vi "swerve_periodic_trajlib.vi"(11 "in ModuleStates":T1[](array[typedef]) {"Angle"."SIN" format="%13.4f"; "Angle"."COS" format="%13.4f"; "Angle"."VALUE" format="%13.4f"}) -> ()   [LabVIEW 2020]
uses:
  <vilib>/Rock Robotics/WPI/ThirdParty/JAS_Junk/TrajLib/SWERVE_DRIVE_MODULE_STATE.ctl
  <vilib>/Rock Robotics/WPI/ThirdParty/JAS_Junk/TrajLib/ROTATION2D.ctl
  <vilib>/Rock Robotics/WPI/ThirdParty/Phoenix-LabVIEW/Motor Controller/Controls/CTRE_Phoenix_MotorControl_ControlMode.ctl
  <vilib>/Rock Robotics/WPI/ThirdParty/JAS_Junk/TrajLib/Conv_Radians_Deg.vi
  swerve_globals.vi
  <vilib>/Rock Robotics/WPI/ThirdParty/Phoenix-LabVIEW/Motor Controller/Get/CTRE_Phoenix_MotorController_GetSelectedSensorData.vi
  TitanLib/Lib/TitanLib.lvlib
  <vilib>/Rock Robotics/WPI/ThirdParty/JAS_Junk/TrajLib/Trajectory_Library.lvlib
panel:
  in  "Drive Motor Constants":T3
  in  "Set Drive Constants":bool
  in  "Set Azimuth Constants":bool
  in  "Azimuth Constants":T3
  out "Pose Estimation (in)":cluster{"Pose[0]":dbl, "Pose[1]":dbl}[](graph)
  in  "wheel offset (in)":dbl format="%_6g"
  in  "Reset Odometry?":bool
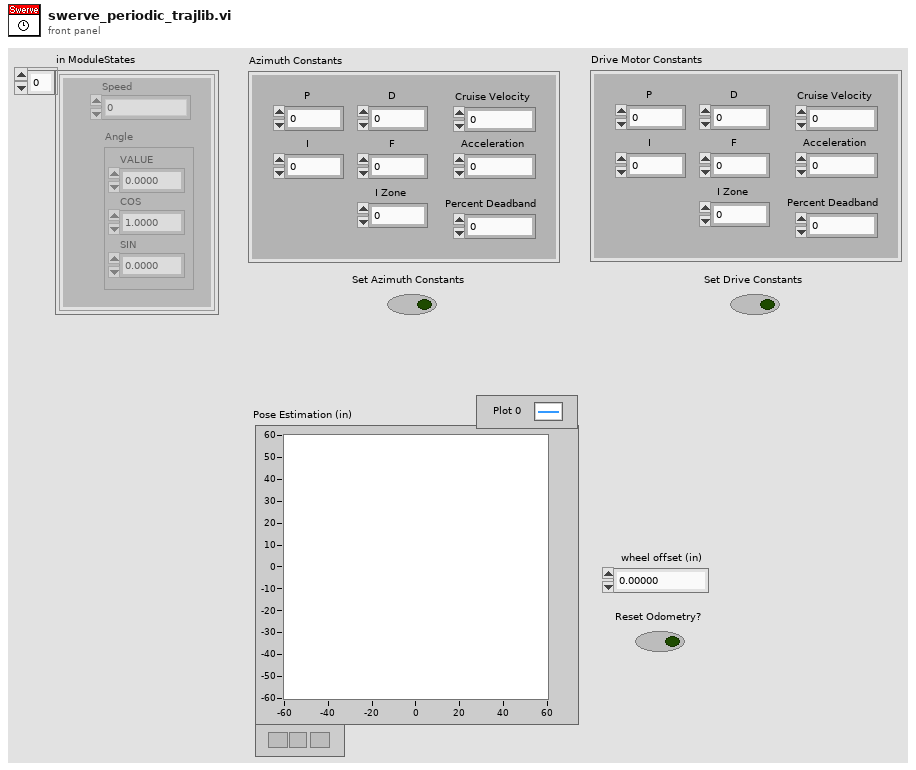
[diagram p1: front panel]
types:
  T1 = typedef "Trajectory_Library.lvlib/SWERVE_DRIVE_MODULE_STATE.ctl" = cluster{"Speed":dbl, "Angle":T2}
  T2 = typedef "Trajectory_Library.lvlib/ROTATION2D.ctl" = cluster{"VALUE":dbl, "COS":dbl, "SIN":dbl}
  T3 = cluster{"P":dbl, "I":dbl, "D":dbl, "F":dbl, "I Zone":dbl, "Cruise Velocity":i32, "Acceleration":i32, "Percent Deadband":dbl}
  T4 = typedef "CTRE_Phoenix_MotorControl_ControlMode.ctl" = u16
  T5 = typedef "WPI_MotorControlDeviceRef.ctl" = cluster{"DeviceStatus":errorcluster, "Type":T6, "PWM":cluster{"PWM Channel":T7, "DeadBand":T8}, "CAN":cluster{"Device Number":u8, "SetOutput VI Ref":variant, "GetOutput VI Ref":variant, "Enable VI Ref":variant, "Disable VI Ref":variant, "Data":variant}, "Invert":bool, "DIO PWM":cluster{"PWM \"Enable\" Channel":T7, "DIOChannel":T9, "PWM Rate":dbl}}
  T6 = typedef "WPI_MotorControlType.ctl" = enum16{"PWM", "CAN", "DIO PWM"}
  T7 = typedef "FPGA_DIOPWMChannel.ctl" = enum8{"PWM 0", "PWM 1", "PWM 2", "PWM 3", "PWM 4", "PWM 5", "PWM 6", "PWM 7", "PWM 8", "PWM 9", "PWM MXP 0", "PWM MXP 1", "PWM MXP 2", "PWM MXP 3", "PWM MXP 4", "PWM MXP 5", "PWM MXP 6", "PWM MXP 7", "PWM MXP 8", "PWM MXP 9", "Invalid"}
  T8 = typedef "WPI_PWMDeadband.ctl" = cluster{"Name":string, "maxPositivePwm":i32, "minPositivePwm":i32, "centerPwm":i32, "maxNegativePwm":i32, "minNegativePwm":i32, "angularRange":u16}
  T9 = typedef "FPGA_DIOChannel.ctl" = enum8{"DIO 0", "DIO 1", "DIO 2", "DIO 3", "DIO 4", "DIO 5", "DIO 6", "DIO 7", "DIO 8", "DIO 9", "DIO MXP 0", "DIO MXP 1", "DIO MXP 2", "DIO MXP 3", "DIO MXP 4", "DIO MXP 5", "DIO MXP 6", "DIO MXP 7", "DIO MXP 8", "DIO MXP 9", "DIO MXP 10", "DIO MXP 11", "DIO MXP 12", "DIO MXP 13", "DIO MXP 14", "DIO MXP 15", "SPI Port CS1", "SPI Port CS2", "SPI Port CS3", "SPI Port MISO", "SPI Port MOSI", "Invalid"}
  T10 = typedef "NI_Matrix.lvlib/RealMatrix.ctl" = dbl[][]
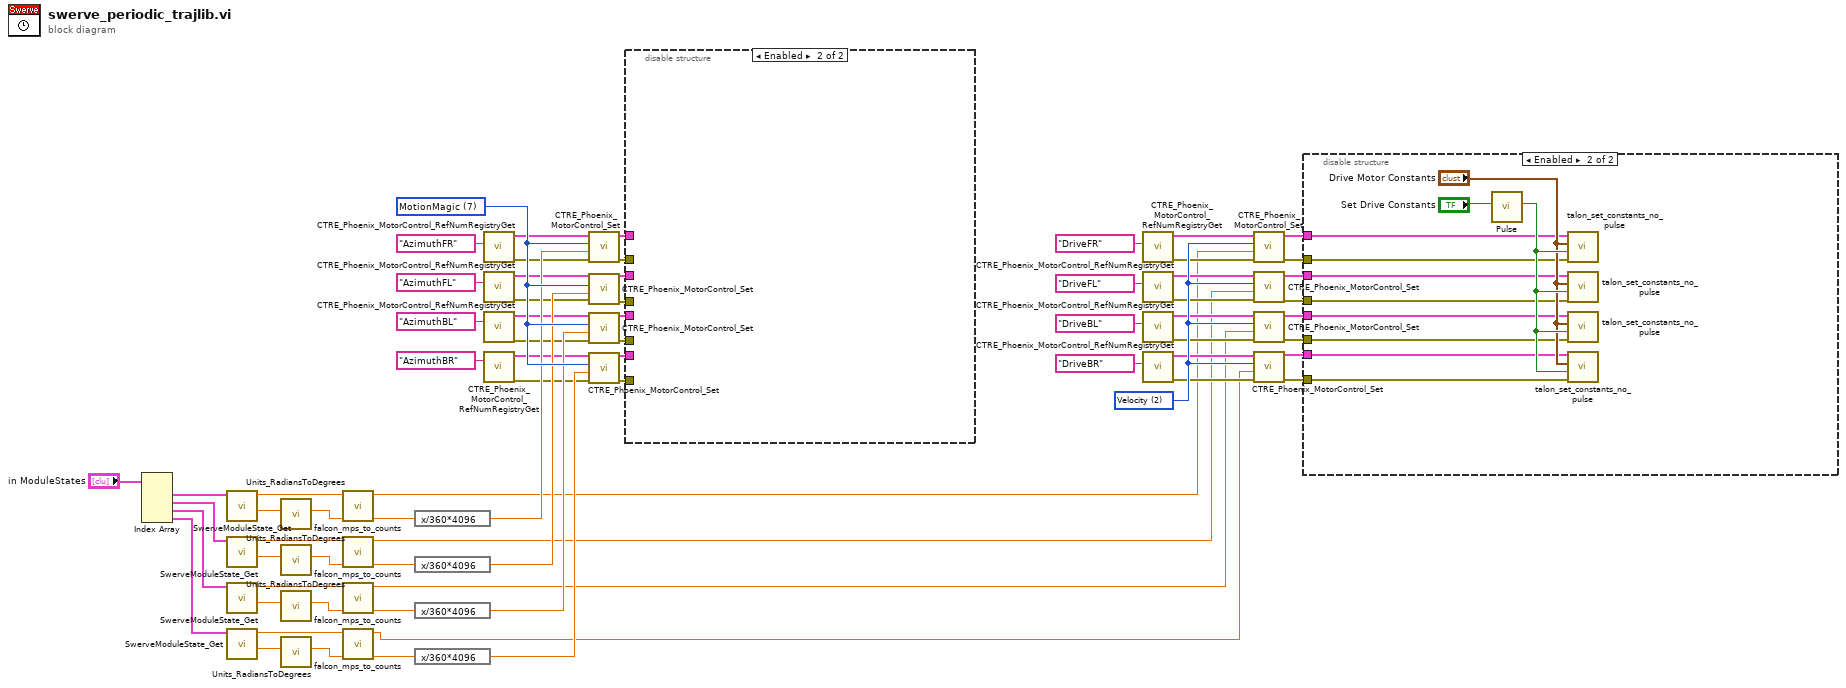
[diagram p0: block diagram]
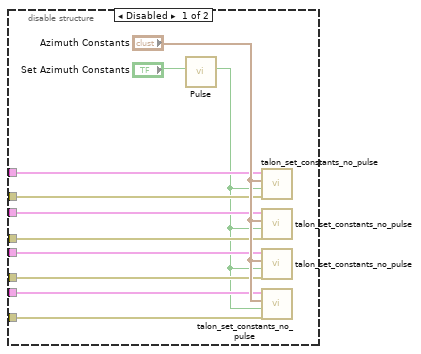
[diagram p2: hidden frame]
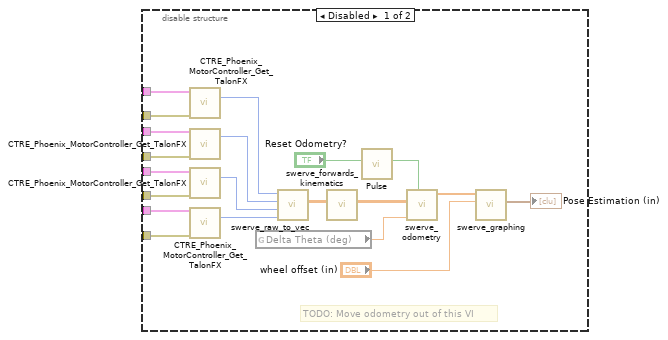
[diagram p3: hidden frame]
diagram:
  w62 = T4 2 items=["PercentOutput"=0, "Position"=1, "Velocity"=2, "Current"=3, "Follower"=5, "MotionProfile"=6, "MotionMagic"=7, "MotionProfileArc"=10, "Disabled"=15] ("Control Mode")
  w67 = T4 7 items=["PercentOutput"=0, "Position"=1, "Velocity"=2, "Current"=3, "Follower"=5, "MotionProfile"=6, "MotionMagic"=7, "MotionProfileArc"=10, "Disabled"=15] ("Control Mode")
  n1 = Index Array(array="in ModuleStates") -> (element #1=w5:T1, element #2=w3:T1, element #3=w2:T1, element #4=w1:T1)  [unwired: 4 in]
  n2 = call <vilib>:"SwerveModuleState_Get.vi"("Desired State"=w5) -> ("Angle RADIANS"=w21:dbl, "Speed M/S"=w14:dbl)  [unwired: 9 in]
  n3 = call <vilib>:"SwerveModuleState_Get.vi"("Desired State"=w3) -> ("Angle RADIANS"=w18:dbl, "Speed M/S"=w15:dbl)  [unwired: 9 in]
  n4 = call <vilib>:"SwerveModuleState_Get.vi"("Desired State"=w2) -> ("Angle RADIANS"=w19:dbl, "Speed M/S"=w16:dbl)  [unwired: 9 in]
  n5 = call <vilib>:"SwerveModuleState_Get.vi"("Desired State"=w1) -> ("Angle RADIANS"=w20:dbl, "Speed M/S"=w17:dbl)  [unwired: 9 in]
  n6 = call <vilib>:"Units_RadiansToDegrees.vi"("Radians"=w21) -> ("Degrees"=w13:dbl)  [unwired: 10 in]
  n7 = call <vilib>:"Units_RadiansToDegrees.vi"("Radians"=w18) -> ("Degrees"=w12:dbl)  [unwired: 10 in]
  n8 = call <vilib>:"Units_RadiansToDegrees.vi"("Radians"=w19) -> ("Degrees"=w11:dbl)  [unwired: 10 in]
  n9 = call <vilib>:"Units_RadiansToDegrees.vi"("Radians"=w20) -> ("Degrees"=w10:dbl)  [unwired: 10 in]
  n10 = call "falcon_mps_to_counts.vi"("Velocity (m/s)"=w14) -> ("Velocity (Counts/100ms)"=w9:dbl)  [unwired: 10 in]
  n11 = call "falcon_mps_to_counts.vi"("Velocity (m/s)"=w15) -> ("Velocity (Counts/100ms)"=w8:dbl)  [unwired: 10 in]
  n12 = call "falcon_mps_to_counts.vi"("Velocity (m/s)"=w16) -> ("Velocity (Counts/100ms)"=w7:dbl)  [unwired: 10 in]
  n13 = call "falcon_mps_to_counts.vi"("Velocity (m/s)"=w17) -> ("Velocity (Counts/100ms)"=w6:dbl)  [unwired: 10 in]
  n14 = expression code="x/360*4096"(w13) -> (w66:dbl)
  n15 = expression code="x/360*4096"(w12) -> (w65:dbl)
  n16 = expression code="x/360*4096"(w11) -> (w64:dbl)
  n17 = expression code="x/360*4096"(w10) -> (w63:dbl)
  n18 = call <vilib>:"CTRE_Phoenix_MotorControl_RefNumRegistryGet.vi"("refnum name"="AzimuthFR") -> ("error out"=w48:errorcluster, "PhoenixMotorControlDevRef"=w49:T5)  [unwired: 9 in]
  n19 = call <vilib>:"CTRE_Phoenix_MotorControl_RefNumRegistryGet.vi"("refnum name"="AzimuthFL") -> ("error out"=w46:errorcluster, "PhoenixMotorControlDevRef"=w47:T5)  [unwired: 9 in]
  n20 = call <vilib>:"CTRE_Phoenix_MotorControl_RefNumRegistryGet.vi"("refnum name"="AzimuthBL") -> ("error out"=w44:errorcluster, "PhoenixMotorControlDevRef"=w45:T5)  [unwired: 9 in]
  n21 = call <vilib>:"CTRE_Phoenix_MotorControl_RefNumRegistryGet.vi"("refnum name"="AzimuthBR") -> ("error out"=w42:errorcluster, "PhoenixMotorControlDevRef"=w43:T5)  [unwired: 9 in]
  n22 = call <vilib>:"CTRE_Phoenix_MotorControl_Set.vi"("error in (no error)"=w48, "Output"=w66, "Control Mode"=w67, "PhoenixMotorControlDevRef"=w49) -> ("error out"=w28:errorcluster, "PhoenixMotorControlDevRef"=w29:T5)  [unwired: 6 in]
  n23 = call <vilib>:"CTRE_Phoenix_MotorControl_Set.vi"("error in (no error)"=w46, "Output"=w65, "Control Mode"=w67, "PhoenixMotorControlDevRef"=w47) -> ("error out"=w26:errorcluster, "PhoenixMotorControlDevRef"=w27:T5)  [unwired: 6 in]
  n24 = call <vilib>:"CTRE_Phoenix_MotorControl_Set.vi"("error in (no error)"=w44, "Output"=w64, "Control Mode"=w67, "PhoenixMotorControlDevRef"=w45) -> ("error out"=w24:errorcluster, "PhoenixMotorControlDevRef"=w25:T5)  [unwired: 6 in]
  n25 = call <vilib>:"CTRE_Phoenix_MotorControl_Set.vi"("error in (no error)"=w42, "Output"=w63, "Control Mode"=w67, "PhoenixMotorControlDevRef"=w43) -> ("error out"=w22:errorcluster, "PhoenixMotorControlDevRef"=w23:T5)  [unwired: 6 in]
  n26 = disable-structure shown="Enabled" {
    disable-tunnel: w29 -> [w77 _]
    disable-tunnel: w28 -> [w76 _]
    disable-tunnel: w27 -> [w75 _]
    disable-tunnel: w26 -> [w74 _]
    disable-tunnel: w25 -> [w73 _]
    disable-tunnel: w24 -> [w72 _]
    disable-tunnel: w23 -> [w71 _]
    disable-tunnel: w22 -> [w70 _]
    frame Disabled {
      n27 = call "Pulse.vi"("Input"="Set Azimuth Constants") -> ("Output"=w68:bool)  [unwired: 10 in]
      n28 = call "talon_set_constants_no_pulse.vi"("error in"=w76, "Set Constants"=w68, "Constants"="Azimuth Constants", "PhoenixMotorControlDevRef"=w77) -> ()  [unwired: 6 in, 2 out]
      n29 = call "talon_set_constants_no_pulse.vi"("error in"=w74, "Set Constants"=w68, "Constants"="Azimuth Constants", "PhoenixMotorControlDevRef"=w75) -> ()  [unwired: 6 in, 2 out]
      n30 = call "talon_set_constants_no_pulse.vi"("error in"=w72, "Set Constants"=w68, "Constants"="Azimuth Constants", "PhoenixMotorControlDevRef"=w73) -> ()  [unwired: 6 in, 2 out]
      n31 = call "talon_set_constants_no_pulse.vi"("error in"=w70, "Set Constants"=w68, "Constants"="Azimuth Constants", "PhoenixMotorControlDevRef"=w71) -> ()  [unwired: 6 in, 2 out]
    }
    frame Enabled {
    }
  }
  n32 = call <vilib>:"CTRE_Phoenix_MotorControl_RefNumRegistryGet.vi"("refnum name"="DriveFR") -> ("error out"=w30:errorcluster, "PhoenixMotorControlDevRef"=w31:T5)  [unwired: 9 in]
  n33 = call <vilib>:"CTRE_Phoenix_MotorControl_RefNumRegistryGet.vi"("refnum name"="DriveFL") -> ("error out"=w32:errorcluster, "PhoenixMotorControlDevRef"=w33:T5)  [unwired: 9 in]
  n34 = call <vilib>:"CTRE_Phoenix_MotorControl_RefNumRegistryGet.vi"("refnum name"="DriveBL") -> ("error out"=w34:errorcluster, "PhoenixMotorControlDevRef"=w35:T5)  [unwired: 9 in]
  n35 = call <vilib>:"CTRE_Phoenix_MotorControl_RefNumRegistryGet.vi"("refnum name"="DriveBR") -> ("error out"=w36:errorcluster, "PhoenixMotorControlDevRef"=w37:T5)  [unwired: 9 in]
  n36 = call <vilib>:"CTRE_Phoenix_MotorControl_Set.vi"("error in (no error)"=w30, "Output"=w9, "Control Mode"=w62, "PhoenixMotorControlDevRef"=w31) -> ("error out"=w60:errorcluster, "PhoenixMotorControlDevRef"=w61:T5)  [unwired: 6 in]
  n37 = call <vilib>:"CTRE_Phoenix_MotorControl_Set.vi"("error in (no error)"=w32, "Output"=w8, "Control Mode"=w62, "PhoenixMotorControlDevRef"=w33) -> ("error out"=w58:errorcluster, "PhoenixMotorControlDevRef"=w59:T5)  [unwired: 6 in]
  n38 = call <vilib>:"CTRE_Phoenix_MotorControl_Set.vi"("error in (no error)"=w34, "Output"=w7, "Control Mode"=w62, "PhoenixMotorControlDevRef"=w35) -> ("error out"=w56:errorcluster, "PhoenixMotorControlDevRef"=w57:T5)  [unwired: 6 in]
  n39 = call <vilib>:"CTRE_Phoenix_MotorControl_Set.vi"("error in (no error)"=w36, "Output"=w6, "Control Mode"=w62, "PhoenixMotorControlDevRef"=w37) -> ("error out"=w54:errorcluster, "PhoenixMotorControlDevRef"=w55:T5)  [unwired: 6 in]
  n40 = disable-structure shown="Enabled" {
    disable-tunnel: w61 -> [w98 w106]
    disable-tunnel: w60 -> [w97 w105]
    disable-tunnel: w59 -> [w96 w104]
    disable-tunnel: w58 -> [w95 w103]
    disable-tunnel: w57 -> [w94 w99]
    disable-tunnel: w56 -> [w93 w102]
    disable-tunnel: w55 -> [w92 w101]
    disable-tunnel: w54 -> [w91 w100]
    frame Disabled {
      # "TODO: Move odometry out of this VI"
      n41 = call-poly <vilib>:"CTRE_Phoenix_MotorController_Get_TalonFX.vi"("PhoenixMotorControlDevRef"=w98, "error in"=w97) -> ("Position (Raw Sensor Units)"=w89:i32)  [unwired: 10 in, 3 out]
      n42 = call-poly <vilib>:"CTRE_Phoenix_MotorController_Get_TalonFX.vi"("PhoenixMotorControlDevRef"=w96, "error in"=w95) -> ("Position (Raw Sensor Units)"=w88:i32)  [unwired: 10 in, 3 out]
      n43 = call-poly <vilib>:"CTRE_Phoenix_MotorController_Get_TalonFX.vi"("PhoenixMotorControlDevRef"=w94, "error in"=w93) -> ("Position (Raw Sensor Units)"=w87:i32)  [unwired: 10 in, 3 out]
      n44 = call-poly <vilib>:"CTRE_Phoenix_MotorController_Get_TalonFX.vi"("PhoenixMotorControlDevRef"=w92, "error in"=w91) -> ("Position (Raw Sensor Units)"=w82:i32)  [unwired: 10 in, 3 out]
      n45 = global read "swerve_globals.vi" "Delta Theta (deg)"() -> (w83:dbl)
      n46 = call "swerve_raw_to_vec.vi"("Raw Position BR"=w82, "Raw Position BL"=w87, "Raw Position FL"=w88, "Raw Position FR"=w89) -> ("Output Vector"=w81:T10)  [unwired: 7 in]
      n47 = call "swerve_forwards_kinematics.vi"("Input Vector"=w81) -> ("Output Vector"=w86:T10)  [unwired: 10 in]
      n48 = call "Pulse.vi"("Input"="Reset Odometry?") -> ("Output"=w79:bool)  [unwired: 10 in]
      n49 = call "swerve_odometry.vi"("Reset?"=w79, "Delta Theta (deg)"=w83, "input vector"=w86) -> ("Pose"=w85:dbl[])  [unwired: 8 in]
      n50 = call "swerve_graphing.vi"("wheel offset"="wheel offset (in)", "Pose"=w85) -> ("Output"=→"Pose Estimation (in)":cluster{"x out":dbl, "y out":dbl}[])  [unwired: 9 in]
    }
    frame Enabled {
      n51 = call "Pulse.vi"("Input"="Set Drive Constants") -> ("Output"=w109:bool)  [unwired: 10 in]
      n52 = call "talon_set_constants_no_pulse.vi"("error in"=w105, "Set Constants"=w109, "Constants"="Drive Motor Constants", "PhoenixMotorControlDevRef"=w106) -> ()  [unwired: 6 in, 2 out]
      n53 = call "talon_set_constants_no_pulse.vi"("error in"=w103, "Set Constants"=w109, "Constants"="Drive Motor Constants", "PhoenixMotorControlDevRef"=w104) -> ()  [unwired: 6 in, 2 out]
      n54 = call "talon_set_constants_no_pulse.vi"("error in"=w102, "Set Constants"=w109, "Constants"="Drive Motor Constants", "PhoenixMotorControlDevRef"=w99) -> ()  [unwired: 6 in, 2 out]
      n55 = call "talon_set_constants_no_pulse.vi"("error in"=w100, "Set Constants"=w109, "Constants"="Drive Motor Constants", "PhoenixMotorControlDevRef"=w101) -> ()  [unwired: 6 in, 2 out]
    }
  }
